vi "Append Command.vi"(8 "error in (no error)":errorcluster, 10 "New Command":string, 11 "ITX Commands in":refnum<class "ITX Commands.lvclass">) -> (0 "error out":errorcluster, 3 "ITX Commands out":refnum<class "ITX Commands.lvclass">)   [LabVIEW 2019, in "ITX Commands.lvclass"]
uses:
  ITX Commands.lvclass
  ITX Commands.lvclass/ITX Commands.ctl
panel:
  out "Command String":string
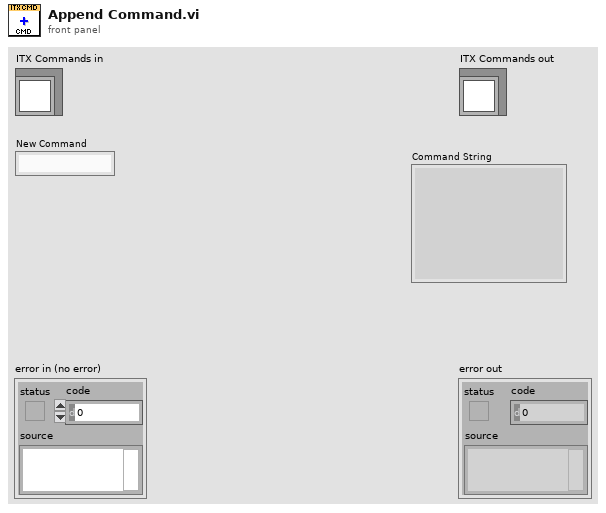
[diagram p1: front panel]
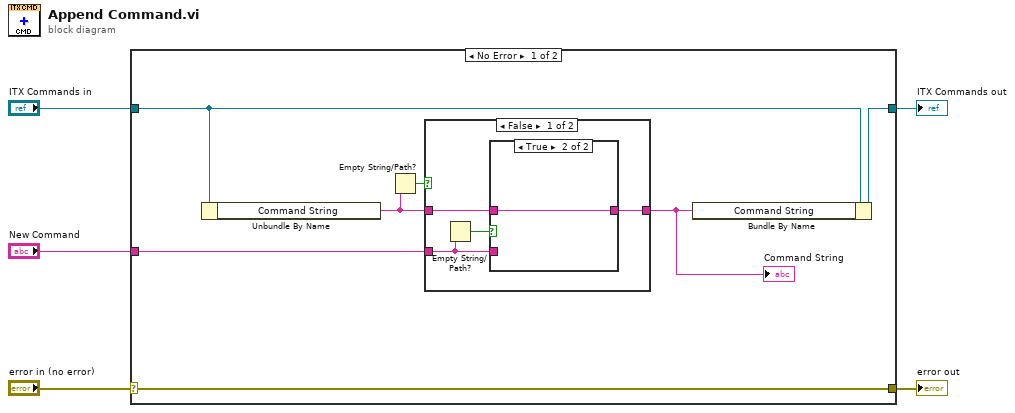
[diagram p0: block diagram]
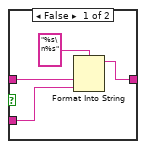
[diagram p2: hidden frame]
diagram:
  n1 = case shown="No Error" "error in (no error)" {
    selector: "error in (no error)" -> [w11 w24]
    tunnel: [w11 w24] -> w4
    tunnel: [w12 w23] -> w2
    tunnel: "ITX Commands in" -> [w9 w23]
    tunnel: "New Command" -> [w8 _]
    frame No Error {
      n2 = Unbundle By Name(w9) -> ("Command String"=w6:string)
      n3 = Empty String/Path?(string/path=w6) -> (empty?=w7:bool)
      n4 = case shown="False" w7 {
        tunnel: [w16 w22] -> w10
        tunnel: w8 -> [w14 w22]
        tunnel: w6 -> [w15 _]
        frame False {
          n5 = Empty String/Path?(string/path=w14) -> (empty?=w13:bool)
          n6 = case shown="True" w13 {
            tunnel: [w19 w21] -> w16
            tunnel: w14 -> [w18 _]
            tunnel: w15 -> [w17 w21]
            frame False {
              n7 = Format Into String(format string="%s\n%s", w17, w18) -> (resulting string=w19:string)  [unwired: 2 in, 1 out]
            }
            frame True {
            }
          }
        }
        frame True {
        }
      }
      "Command String" <- w10
      n8 = Bundle By Name(cluster=w9, "Command String"=w10) -> (w12:refnum<class "ITX Commands.lvclass">)
    }
    frame Error {
    }
  }
  "error out" <- w4
  "ITX Commands out" <- w2
